vi "Logging_Engine.vi"(1 "Test Name":string caption="String", 2 "queue":refnum<queue>, 3 "notifier out":refnum<notifier>) -> ()   [LabVIEW 2018]
uses:
  Notifier_control.ctl
  cluster_enum.ctl
  <vilib>/Utility/error.llb/DialogType.ctl
  <vilib>/Waveform/WDTOps.llb/WDT Get Waveform Time Array DBL.vi
panel:
  out "Save Path":path caption="Path"
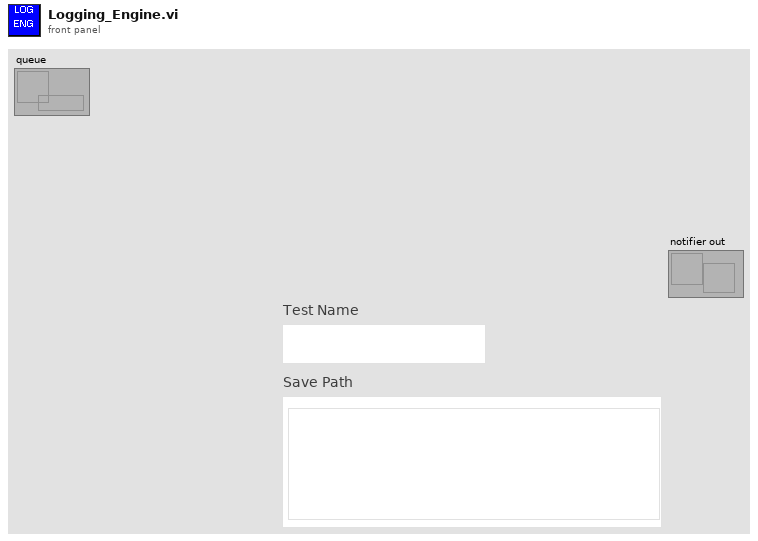
[diagram p1: front panel]
types:
  T1 = typedef "Notifier_control.ctl" = enum16{"Quit", "Run", "Tare", "Save"}
  T2 = typedef "DialogType.ctl" = u16
  T3 = enum16{"open", "open or create", "create or replace", "create", "open (read-only)"}
  T4 = typedef "cluster_enum.ctl" = enum16{"Card 2 Tared", "Card 2", "Card 1 Tared", "Card 1"}
  T5 = cluster{"C Module":T4, " Data":waveform(dbl)[], string[]}
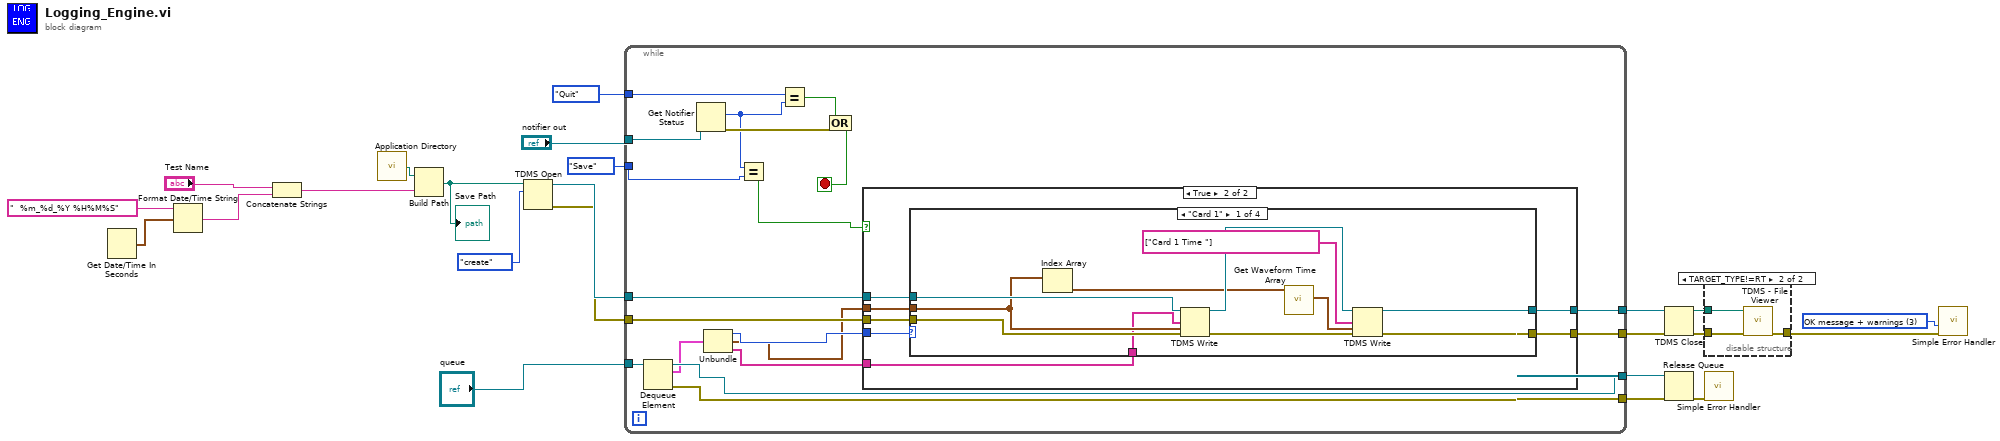
[diagram p0: block diagram]
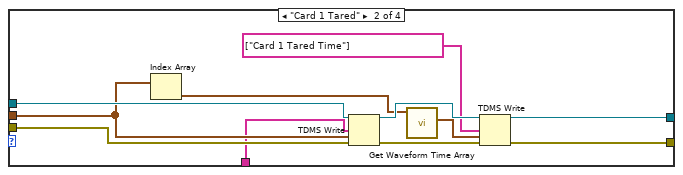
[diagram p4: hidden frame]
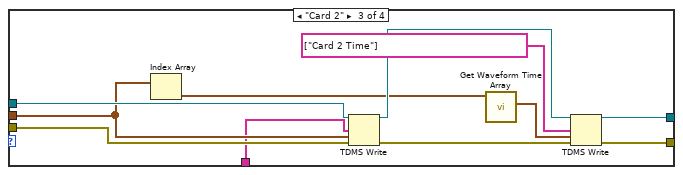
[diagram p5: hidden frame]
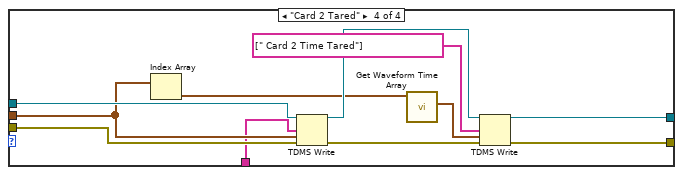
[diagram p6: hidden frame]
diagram:
  w13 = T2 3 items=["no dialog", "OK message", "continue or stop message", "OK message + warnings", "continue/stop + warnings"] ("type of dialog (OK msg:1)")
  n1 = Get Date/Time In Seconds() -> (seconds since 1Jan1904=w22:timestamp)
  n2 = Format Date/Time String(time format string (%c)="  %m_%d_%Y %H%M%S", seconds (now)=w22) -> (date/time string=w19:string)  [unwired: 1 in]
  n3 = Concatenate Strings("Test Name", w19) -> (w18:string)
  n4 = call <vilib>:"Application Directory.vi"() -> ("Application Directory"=w20:path)
  n5 = Build Path(base path=w20, name or relative path=w18) -> (appended path=w17:path)
  "Save Path" <- w17
  n6 = TDMS Open(10:T3."create" ("operation"), 11:w17) -> (0:w14:errorcluster, 3:w15:refnum<k34>)  [unwired: 5 in]
  n7 = while {
    tunnel: w15 -> [w42]
    tunnel: w14 -> [w41]
    tunnel: [w40] -> w9
    tunnel: [w39] -> w8
    tunnel: [w28] -> w6
    tunnel: [w29] -> w5
    tunnel: "notifier out" -> [w38]
    tunnel: Notifier_control."Quit" -> [w37]
    tunnel: Notifier_control."Save" -> [w33]
    tunnel: "queue" -> [w30]
    stop <- w34 stop-if-true
    n8 = Dequeue Element(queue=w30) -> (queue out=w28:refnum<queue>, element=w26:T5, error out=w29:errorcluster)  [unwired: 2 in, 1 out]
    n9 = Get Notifier Status(notifier=w38) -> (current notification=w32:T1, error out=w36:errorcluster)  [unwired: 1 in, 3 out]
    n10 = Unbundle(w26) -> ("C Module"=w25:T4, "Data"=w24:waveform(dbl)[], w27:string[])
    n11 = Equal?(x=w32, y=w33) -> (x = y?=w31:bool)
    n12 = Equal?(x=w37, y=w32) -> (x = y?=w35:bool)
    n13 = Compound Arithmetic op=OR(w35, w36) -> (w34:bool)
    n14 = case shown="True" w31 {
      tunnel: w25 -> [_ w51]
      tunnel: w42 -> [w44 w50]
      tunnel: w41 -> [w43 w49]
      tunnel: w24 -> [_ w48]
      tunnel: [w44 w47] -> w40
      tunnel: [w43 w46] -> w39
      tunnel: w27 -> [_ w45]
      frame False {
      }
      frame True {
        n15 = case shown="\"Card 1\"" w51 {
          tunnel: w50 -> [w62 w73 w84 w95]
          tunnel: w49 -> [w61 w72 w83 w94]
          tunnel: w48 -> [w55 w66 w75 w86]
          tunnel: [w57 w68 w79 w90] -> w47
          tunnel: [w58 w69 w80 w91] -> w46
          tunnel: w45 -> [w52 w63 w74 w85]
          frame "Card 1" {
            n16 = Index Array(array=w55) -> (element=w54:waveform(dbl))  [unwired: 1 in]
            n17 = TDMS Write(0:w62, 7:w52, 9:w55, 11:w61) -> (4:w60:refnum<k34>, 15:w59:errorcluster)  [unwired: 2 in, 2 out]
            n18 = call-poly <vilib>:"Get Waveform Time Array.vi"("waveform in"=w54) -> ("X array"=w53:timestamp[])  [unwired: 9 in, 1 out]
            n19 = TDMS Write(0:w60, 7:string[] ["Card 1 Time "] ("channel name(s) in (Untitled)"), 9:w53, 11:w59) -> (4:w57:refnum<k34>, 15:w58:errorcluster)  [unwired: 2 in, 2 out]
          }
          frame "Card 1 Tared" {
            n20 = Index Array(array=w66) -> (element=w65:waveform(dbl))  [unwired: 1 in]
            n21 = TDMS Write(0:w73, 7:w63, 9:w66, 11:w72) -> (4:w71:refnum<k34>, 15:w70:errorcluster)  [unwired: 2 in, 2 out]
            n22 = call-poly <vilib>:"Get Waveform Time Array.vi"("waveform in"=w65) -> ("X array"=w64:timestamp[])  [unwired: 9 in, 1 out]
            n23 = TDMS Write(0:w71, 7:string[] ["Card 1 Tared Time"] ("channel name(s) in (Untitled)"), 9:w64, 11:w70) -> (4:w68:refnum<k34>, 15:w69:errorcluster)  [unwired: 2 in, 2 out]
          }
          frame "Card 2" {
            n24 = Index Array(array=w75) -> (element=w77:waveform(dbl))  [unwired: 1 in]
            n25 = TDMS Write(0:w84, 7:w74, 9:w75, 11:w83) -> (4:w82:refnum<k34>, 15:w81:errorcluster)  [unwired: 2 in, 2 out]
            n26 = call-poly <vilib>:"Get Waveform Time Array.vi"("waveform in"=w77) -> ("X array"=w76:timestamp[])  [unwired: 9 in, 1 out]
            n27 = TDMS Write(0:w82, 7:string[] ["Card 2 Time"] ("channel name(s) in (Untitled)"), 9:w76, 11:w81) -> (4:w79:refnum<k34>, 15:w80:errorcluster)  [unwired: 2 in, 2 out]
          }
          frame "Card 2 Tared" {
            n28 = Index Array(array=w86) -> (element=w88:waveform(dbl))  [unwired: 1 in]
            n29 = TDMS Write(0:w95, 7:w85, 9:w86, 11:w94) -> (4:w93:refnum<k34>, 15:w92:errorcluster)  [unwired: 2 in, 2 out]
            n30 = call-poly <vilib>:"Get Waveform Time Array.vi"("waveform in"=w88) -> ("X array"=w87:timestamp[])  [unwired: 9 in, 1 out]
            n31 = TDMS Write(0:w93, 7:string[] [" Card 2 Time Tared"] ("channel name(s) in (Untitled)"), 9:w87, 11:w92) -> (4:w90:refnum<k34>, 15:w91:errorcluster)  [unwired: 2 in, 2 out]
          }
        }
      }
    }
  }
  n32 = TDMS Close(8:w8, 11:w9) -> (0:w11:errorcluster, 3:w12:path)
  n33 = Release Queue(queue=w6, error in (no error)=w5) -> (error out=w7:errorcluster)  [unwired: 1 in, 2 out]
  n34 = disable-structure shown="TARGET_TYPE!=RT" {
    disable-tunnel: w11 -> [w96 w99]
    disable-tunnel: w12 -> [_ w98]
    disable-tunnel: [w96 w97] -> w10
    frame condition #0 {
    }
    frame condition #1 (active) {
      n35 = call <vilib>:"TDMS - File Viewer.vi"("error in (no error)"=w99, "file path"=w98) -> ("error out"=w97:errorcluster)  [unwired: 5 out]
    }
  }
  n36 = call <vilib>:"Simple Error Handler.vi"("error in (no error)"=w7) -> ()  [unwired: 1 in, 8 out]
  n37 = call <vilib>:"Simple Error Handler.vi"("type of dialog (OK msg:1)"=w13, "error in (no error)"=w10) -> ()  [unwired: 1 in, 7 out]
